vi "Quary Output Current.vi"(9 "error in (no error)":errorcluster, 10 "VISA resource name":refnum<visa-resource-name>) -> (0 "Output Current(A)":dbl, 1 "error out":errorcluster, 2 "VISA resource name out":refnum<visa-resource-name>)   [LabVIEW 2018]
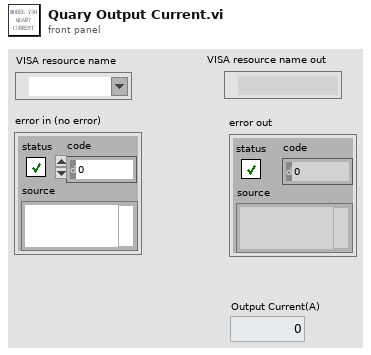
[diagram p1: front panel]
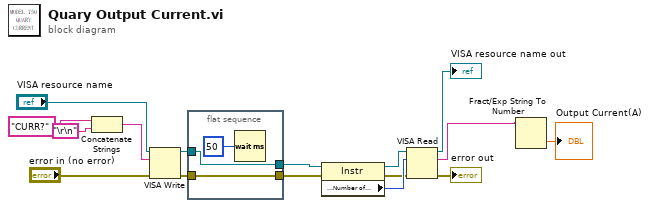
[diagram p0: block diagram]
diagram:
  n1 = Concatenate Strings("CURR?" ("字符串"), "\r\n") -> (w12:string)
  n2 = VISA Write(VISA resource name="VISA resource name", write buffer=w12, error in (no error)="error in (no error)") -> (VISA resource name out=w11:refnum<visa-resource-name>, error out=w10:errorcluster)  [unwired: 1 out]
  n3 = flat-sequence {
    tunnel: [w19] -> w7
    tunnel: w11 -> [w19]
    tunnel: [w18] -> w6
    tunnel: w10 -> [w18]
    frame #0 {
      n4 = Wait (ms)(milliseconds to wait=u32 50 ("等待时间（毫秒）")) -> ()  [unwired: 1 out]
    }
  }
  n5 = property class="Instr"(reference=w7, error in=w6) -> (reference out=w5:refnum<visa-resource-name>, error out=w3:errorcluster, "Serial Settings:Number of Bytes at Serial Port"=w4:u32)
  n6 = VISA Read(VISA resource name=w5, byte count=w4, error in (no error)=w3) -> (VISA resource name out=→"VISA resource name out":refnum<visa-resource-name>, read buffer=w2:string, error out=→"error out":errorcluster)  [unwired: 1 out]
  n7 = Fract/Exp String To Number(string=w2) -> (number=→"Output Current(A)":dbl)  [unwired: 3 in, 1 out]
